vi "Simulator Initialize.vi"(8 "error in (no error)":errorcluster, 11 "Module Name":string) -> (0 "error out":errorcluster, 3 "data value reference":refnum<data-value>)   [LabVIEW 2019, in "ADLINK Motion Card.lvlib"]
uses:
  ADLINK Motion Card.lvlib
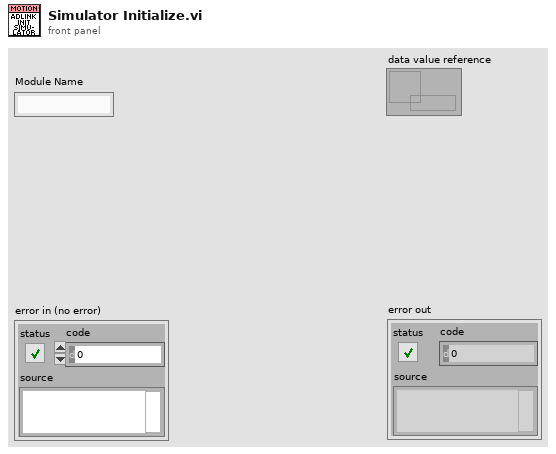
[diagram p1: front panel]
types:
  T1 = cluster{"Current Position":dbl, "Target Position":dbl, "Velocity":dbl, "Acceleration":dbl, "Arrived?":bool}
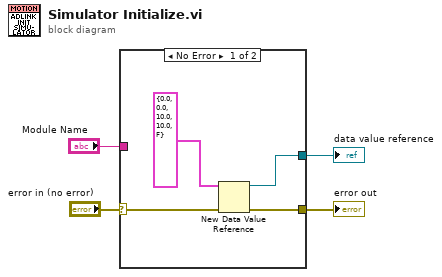
[diagram p0: block diagram]
diagram:
  n1 = case shown="No Error" "error in (no error)" {
    selector: "error in (no error)" -> [w6 w9]
    tunnel: [w8 w9] -> w4
    tunnel: "Module Name" -> [_ _]
    tunnel: [w5 _] -> w1
    frame No Error {
      n2 = New Data Value Reference(data value=T1 {"Current Position"=0.0, "Target Position"=0.0, "Velocity"=10.0, "Acceleration"=10.0, "Arrived?"=FALSE} ("SEQ Data"), error in=w6) -> (data value reference=w5:refnum<data-value>, error out=w8:errorcluster)
    }
    frame Error {
    }
  }
  "error out" <- w4
  "data value reference" <- w1
